vi "Initialize Engine Pointer (U64).vi"(8 "error in (no error)":errorcluster, 9 "size":u64 format="%d bytes", 10 "address":u64 format="%016x", 11 "Framework in":refnum<class "Framework.lvclass">) -> (0 "error out":errorcluster, 3 "Framework out":refnum<class "Framework.lvclass">)   [LabVIEW 2017, in "DSF Core.lvlib" / "Framework.lvclass"]
uses:
  Framework.lvclass
  <vilib>/NI/Memory Manager/Classes/Pointer/Pointer.lvclass
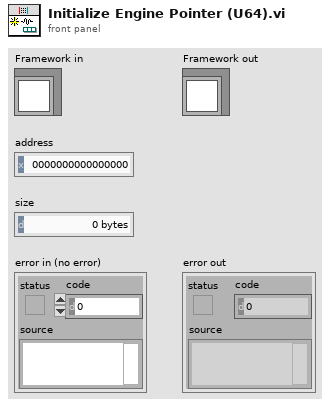
[diagram p1: front panel]
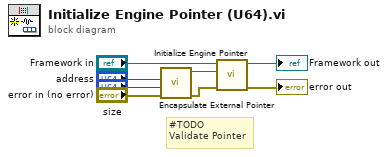
[diagram p0: block diagram]
diagram:
  # "#TODO\nValidate Pointer"
  n1 = call <vilib>:"Encapsulate External Pointer.vi"("error in (no error)"="error in (no error)", "size"="size", "address"="address") -> ("error out"=w3:errorcluster, "Pointer out"=w5:refnum<class "Pointer.lvclass">)  [unwired: 7 in]
  n2 = call "Initialize Engine Pointer.vi"("error in (no error)"=w3, "Engine Pointer"=w5, "Framework in"="Framework in") -> ("error out"=→"error out":errorcluster, "Framework out"=→"Framework out":refnum<class "Framework.lvclass">)  [unwired: 7 in]
